vi "SetTimestamp.vi"(9 "Error in":errorcluster) -> (1 "Error out":errorcluster)   [LabVIEW 2017, in "GPError.lvlib"]
doc: "Sets a timestamp on <B>Error in</B> if it contains an error or warning. If a timestamp is already present it will be replaced with this new timestamp.\n\nIf <B>Error in</B> contains an appended error only the primary error/warning will get a new timestamp from this VI.\n\nThis VI is inlined.\n\nSteen Schmidt\nGPower\n14/11 2014"
uses:
  GPError.lvlib
panel:
  # "Copyright © 2013\nSteen Schmidt, GPower\nSee enclosed license file for terms and conditions"
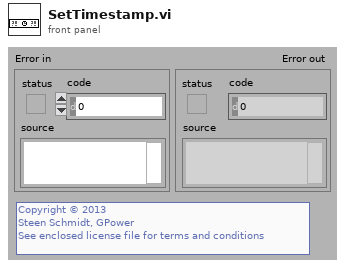
[diagram p1: front panel]
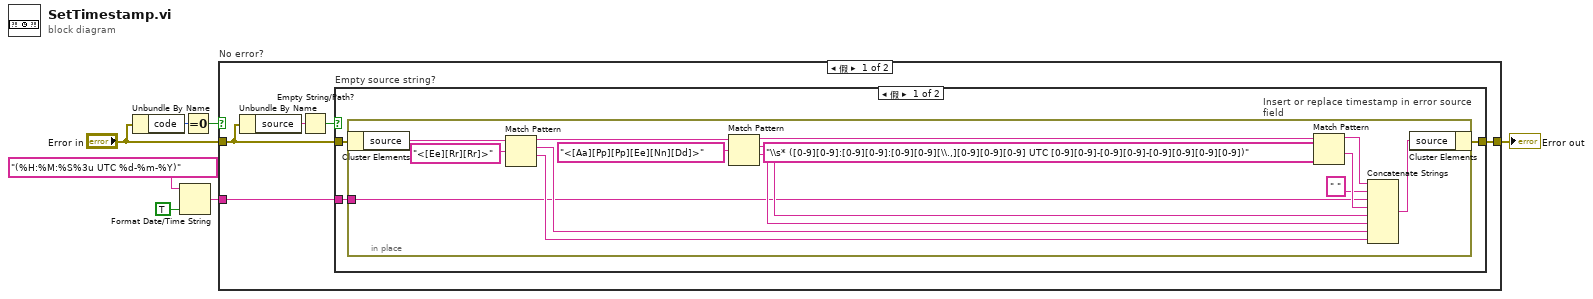
[diagram p0: block diagram]
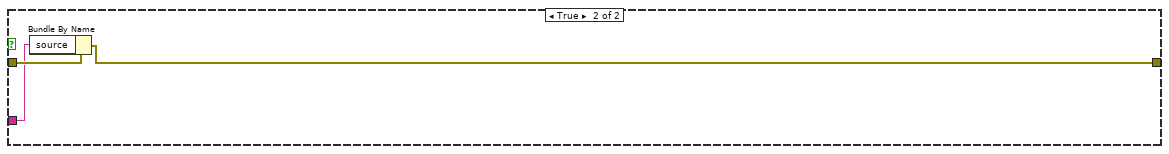
[diagram p2: hidden frame]
diagram:
  n1 = Unbundle By Name("Error in") -> ("code"=w5:i32)
  n2 = Format Date/Time String(time format string (%c)="(%H:%M:%S%3u UTC %d-%m-%Y)", UTC format=TRUE) -> (date/time string=w1:string)  [unwired: 1 in]
  n3 = Equal To 0?(x=w5) -> (x = 0?=w4:bool)
  n4 = case "No error?" shown="假" w4 {
    tunnel: [w12 w34] -> w7
    tunnel: "Error in" -> [w10 w34]
    tunnel: w1 -> [w11 _]
    frame False {
      n5 = Unbundle By Name(w10) -> ("source"=w9:string)
      n6 = Empty String/Path?(string/path=w9) -> (empty?=w8:bool)
      n7 = case "Empty source string?" shown="假" w8 {
        tunnel: [w15 w32] -> w12
        tunnel: w11 -> [w14 w31]
        tunnel: w10 -> [w13 w33]
        frame False {
          n8 = in-place "Insert or replace timestamp in error source field" {
            in-place-border: w14 -> [w19]
            n9 = in-place-cluster #1(w13) -> ("source"=w25:string)
            n10 = Match Pattern(string=w25, regular expression="<[Ee][Rr][Rr]>") -> (before substring=w28:string, match substring=w24:string, after substring=w23:string)  [unwired: 1 in, 1 out]
            n11 = Match Pattern(string=w28, regular expression="<[Aa][Pp][Pp][Ee][Nn][Dd]>") -> (before substring=w26:string, match substring=w21:string, after substring=w22:string)  [unwired: 1 in, 1 out]
            n12 = Match Pattern(string=w26, regular expression="\\s* ([0-9][0-9]:[0-9][0-9]:[0-9][0-9][\\.,][0-9][0-9][0-9] UTC [0-9][0-9]-[0-9][0-9]-[0-9][0-9][0-9][0-9])" ("time format string (%c)")) -> (before substring=w17:string, after substring=w20:string)  [unwired: 1 in, 2 out]
            n13 = Concatenate Strings(w17, " " ("string"), w19, w20, w21, w22, w24, w23) -> (w18:string)
            n14 = in-place-cluster #1("source"=w18) -> (w15:errorcluster)
          }
        }
        frame True {
          n15 = Bundle By Name(cluster=w33, "source"=w31) -> (w32:errorcluster)
        }
      }
    }
    frame True {
    }
  }
  "Error out" <- w7
